vi "UTILITY Modbus 32bit Number Combine.vi"(11 "Holding Registers":u16[](array[numeric]) format="%.0x") -> (2 "word swapped":u32 format="%.0x", 3 "Data":sgl)   [LabVIEW 2018]
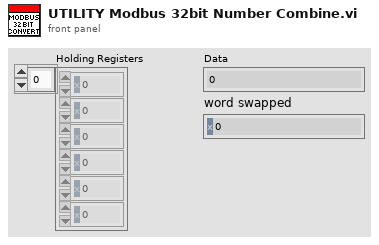
[diagram p1: front panel]
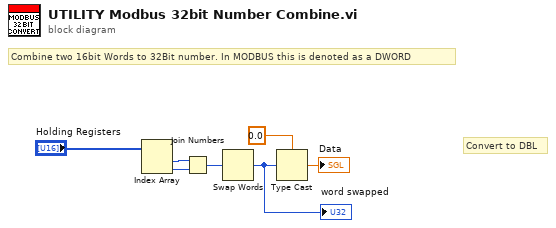
[diagram p0: block diagram]
diagram:
  # "Convert to DBL"
  # "Combine two 16bit Words to 32Bit number. In MODBUS this is denoted as a DWORD"
  n1 = Index Array(array="Holding Registers") -> (element #1=w2:u16, element #2=w4:u16)  [unwired: 2 in]
  n2 = Join Numbers(hi=w2, lo=w4) -> ((hi.lo)=w1:u32)
  n3 = Swap Words(1:w1) -> (0:w3:u32)
  "word swapped" <- w3
  n4 = Type Cast(type=sgl 0.0, x=w3) -> (*(type *) &x=→"Data":sgl)
